vi "Lambda Percentage Flow (Set).vi"(6 "ISOBUS address":T3=-1 caption="ISOBUS address (-1)", 8 "error in":errorcluster, 9 "Unit":T1, 10 "Percentage Open":dbl min=0.0 max=100.0 format="%#.1f", 11 "Mercury Reference In":T5) -> (0 "error out":errorcluster, 2 "Response":T2, 3 "Mercury Reference Out":T5, 4 "Valid?":T4)   [LabVIEW 2013, in "Mercury iXX.lvlib" / "Lambda.lvlib"]
doc: "Set the percentage of the flow output associated with control loop."
uses:
  <instrlib>/Mercury iXX/Public/Libraries/Lambda.lvlib
  <instrlib>/Mercury iXX/Public/Controls/Mercury Reference.ctl
  <instrlib>/Mercury iXX/Public/Controls/Comms Transport Layer.ctl
  <instrlib>/Mercury iXX/Private/Controls/Query Dynamic Reference.ctl
  <instrlib>/Mercury iXX/Public/Controls/Is Valid LED.ctl
  <instrlib>/Mercury iXX/Public/Controls/ISOBus Address.ctl
  <instrlib>/Mercury iXX/Public/Controls/Response String.ctl
  <instrlib>/Mercury iXX/Public/Controls/Unit String.ctl
  <instrlib>/Mercury iXX/Private/Controls/Command Verbs.ctl
  <instrlib>/Mercury iXX/Mercury iXX.lvlib
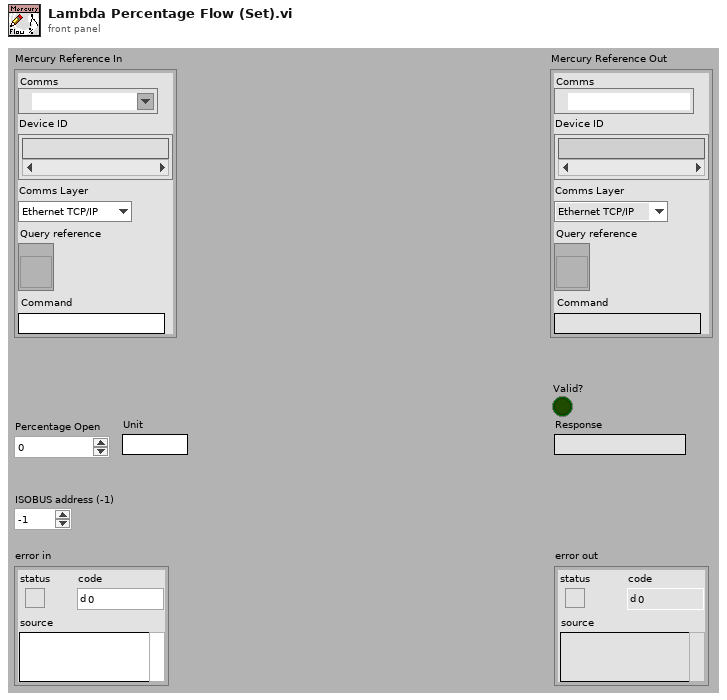
[diagram p1: front panel]
types:
  T1 = typedef "Mercury iXX.lvlib/Unit String.ctl" = string
  T2 = typedef "Mercury iXX.lvlib/Response String.ctl" = string
  T3 = typedef "Mercury iXX.lvlib/ISOBus Address.ctl" = i32
  T4 = typedef "Mercury iXX.lvlib/Is Valid LED.ctl" = bool
  T5 = typedef "Mercury iXX.lvlib/Mercury Reference.ctl" = cluster{"Comms":refnum<visa-resource-name>, "Device ID":string[], "Comms Layer":T6, "Command":string, "Query reference":T7}
  T6 = typedef "Mercury iXX.lvlib/Comms Transport Layer.ctl" = enum16{"Ethernet TCP/IP", "USB", "ISOBus - RS-232", "GPIB"}
  T7 = typedef "Mercury iXX.lvlib/Query Dynamic Reference.ctl" = refnum<vi>
  T8 = typedef "Mercury iXX.lvlib/Command Verbs.ctl" = string
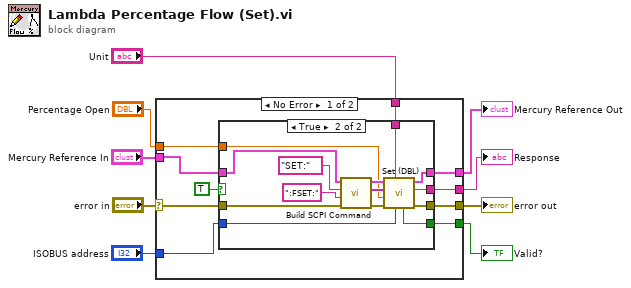
[diagram p0: block diagram]
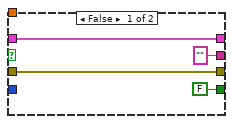
[diagram p2: hidden frame]
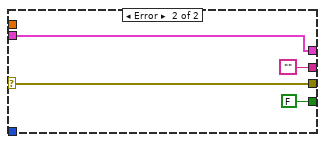
[diagram p3: hidden frame]
diagram:
  n1 = case shown="No Error" "error in" {
    selector: "error in" -> [w10 w40]
    tunnel: "Mercury Reference In" -> [w11 w41]
    tunnel: [w17 w41] -> w5
    tunnel: [w16 w40] -> w2
    tunnel: "ISOBUS address" -> [w18 _]
    tunnel: [w15 ""] -> w4
    tunnel: [w14 FALSE ("Valid?")] -> w3
    tunnel: "Percentage Open" -> [w19 _]
    tunnel: "Unit" -> [w13 _]
    frame No Error {
      n2 = case shown="True" TRUE {
        tunnel: w19 -> [_ w29]
        tunnel: w10 -> [w23 w30]
        tunnel: w18 -> [_ w25]
        tunnel: w11 -> [w22 w33]
        tunnel: [w22 w32] -> w17
        tunnel: [w23 w31] -> w16
        tunnel: [T2 "" ("Response") w27] -> w15
        tunnel: [T4 FALSE ("Valid?") w26] -> w14
        tunnel: w13 -> [_ w24]
        frame False {
        }
        frame True {
          n3 = call <instrlib>:"Build SCPI Command.vi"("error in"=w30, "Noun(s)"=":FSET:" ("Command"), "Verb"=T8 "SET:", "Mercury Reference In"=w33) -> ("error out"=w37:errorcluster, "SCPI Message(s)"=w36:string[], "Mercury Reference Out"=w35:T5)  [unwired: 5 out]
          n4 = call <instrlib>:"Set (DBL).vi"("ISOBUS address"=w25, "Unit"=w24, "error in"=w37, "Command Value (Dbl)"=w29, "SCPI Message(s)"=w36, "Mercury Reference In"=w35) -> ("error out"=w31:errorcluster, "Response"=w27:T2, "Mercury Reference Out"=w32:T5, "Valid?"=w26:T4)  [unwired: 2 out]
        }
      }
    }
    frame Error {
    }
  }
  "Mercury Reference Out" <- w5
  "error out" <- w2
  "Valid?" <- w3
  "Response" <- w4
